vi "TDMS DAQ File Path.vi"(10 "Experiment Name":string, 11 "Operator Name":string) -> (3 "appended path":path)   [LabVIEW 2011]
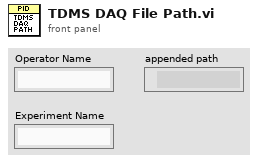
[diagram p1: front panel]
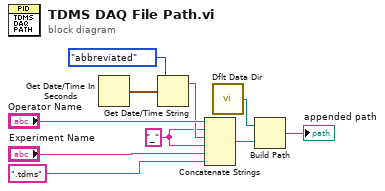
[diagram p0: block diagram]
diagram:
  w3 = "_"
  n1 = Get Date/Time In Seconds() -> (seconds since 1Jan1904=w5:timestamp)
  n2 = Get Date/Time String(date format (0)=enum16{"short", "long", "abbreviated"}."abbreviated", seconds (now)=w5) -> (date string=w4:string)  [unwired: 1 in, 1 out]
  n3 = Concatenate Strings("Operator Name", w3, w4, w3, "Experiment Name", ".tdms" ("string")) -> (w6:string)
  n4 = call <vilib>:"Dflt Data Dir.vi"() -> ("App:Default Data Directory"=w7:path)
  n5 = Build Path(base path=w7, name or relative path=w6) -> (appended path=→"appended path":path)
